vi "Log Target.vi"(8 "error in":errorcluster, 10 "Entry":string, 11 "Study Actor in":refnum<class "Study Actor.lvclass">) -> (0 "error out":errorcluster, 3 "Study Actor out":refnum<class "Study Actor.lvclass">)   [LabVIEW 2023, in "Study Actor.lvlib" / "Study Actor.lvclass"]
uses:
  Study Actor.lvclass
  Study Actor.lvclass/Study Actor.ctl
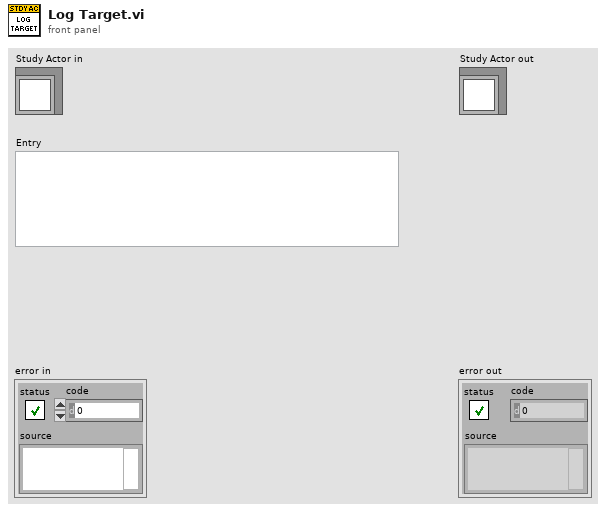
[diagram p1: front panel]
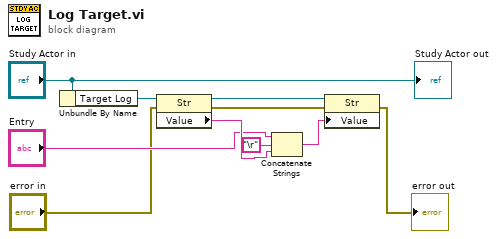
[diagram p0: block diagram]
diagram:
  n1 = Unbundle By Name("Study Actor in") -> ("Target Log"=w9:refnum<vi>)
  n2 = property class="Str"(reference=w9, error in="error in") -> (reference out=w4:refnum<vi>, error out=w3:errorcluster, "Value"=w7:string)
  n3 = Concatenate Strings("Entry", "\r", w7) -> (w2:string)
  n4 = property class="Str"(reference=w4, error in=w3, "Value"=w2) -> (error out=→"error out":errorcluster)  [unwired: 1 out]
  "Study Actor out" <- "Study Actor in"
